vi "Wrapper_Open File+InitPicture.vi"(8 "error in (no error)":errorcluster, 11 "FilePath":path) -> (0 "error out":errorcluster, 2 "LIMPICTUREout":T2, 3 "hFile out":T1, 5 "N Frames (= uiSequenceCount)":u32)   [LabVIEW 2014, in "ND2_Reader_32.lvlib"]
uses:
  ND2_Reader_32.lvlib
  controls/cluster_LIMPICTURE.ctl
  controls/numeric_LIMFILEHANDLE.ctl
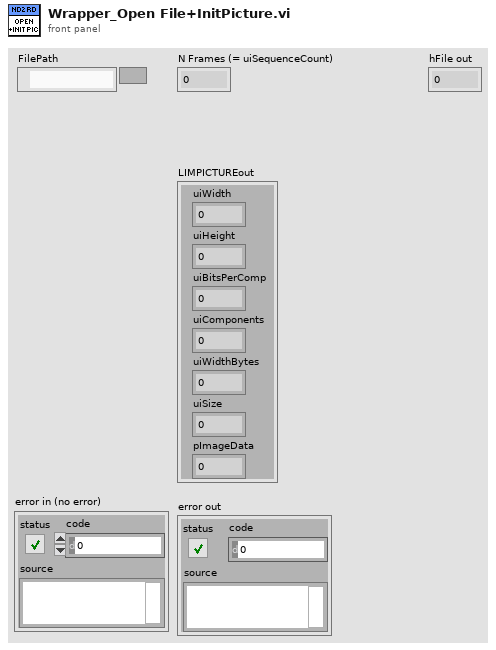
[diagram p1: front panel]
types:
  T1 = typedef "numeric_LIMFILEHANDLE.ctl" = i32
  T2 = typedef "cluster_LIMPICTURE.ctl" = cluster{"uiWidth":u32, "uiHeight":u32, "uiBitsPerComp":u32, "uiComponents":u32, "uiWidthBytes":u32, "uiSize":u32, "pImageData":u32}
  T3 = typedef "cluster_LIMATTRIBUTES.ctl" = cluster{"uiWidth":u32, "uiWidthBytes":u32, "uiHeight":u32, "uiComp":u32, "uiBpcInMemory":u32, "uiBpcSignificant":u32, "uiSequenceCount":u32, "uiTileWidth":u32, "uiTileHeight":u32, "uiCompression":u32, "uiQuality":u16}
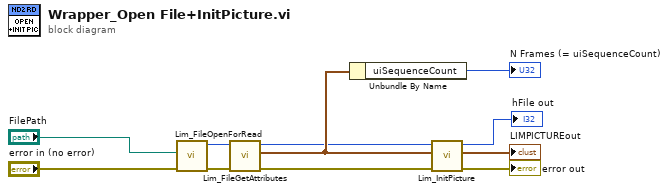
[diagram p0: block diagram]
diagram:
  n1 = call "Lim_FileOpenForRead.vi"("error in (no error)"="error in (no error)", "FilePath"="FilePath") -> ("error out"=w3:errorcluster, "hFile"=w2:T1)  [unwired: 8 in]
  n2 = call "Lim_FileGetAttributes.vi"("error in (no error)"=w3, "hFile in"=w2) -> ("error out"=w4:errorcluster, "LIMATTRIBUTES"=w6:T3, "hFile out"=w5:T1)  [unwired: 5 in, 2 out]
  n3 = Unbundle By Name(w6) -> ("uiSequenceCount"=→"N Frames (= uiSequenceCount)":u32)
  n4 = call "Lim_InitPicture.vi"("error in (no error)"=w4, "LIMATTRIBUTES"=w6, "hFile in"=w5) -> ("error out"=→"error out":errorcluster, "LIMPICTURE"=→"LIMPICTUREout":T2, "hFile out"=→"hFile out":T1)  [unwired: 5 in, 1 out]
